vi "Agilent SNA Set Sweep Time.vi"(4 "Passthrough (T)":bool=TRUE, 6 "Channel":i8=1 min=1 max=99 step=1, 7 "Agilent SNA & SWP":T1, 8 "error in (no error)":errorcluster, 10 "Sweep Time, s (-1: Auto)":dbl=-1.0, 11 "VISA Resource Names":T2) -> (0 "error out":errorcluster, 3 "dup VISA Resource Names":T2)   [LabVIEW 2011]
doc: "This Vi for the HP8753B Network Analyzer is used to set averaging, smoothing, and the IF bandwidth."
uses:
  TypeDefs/Agilent SNA VISA.ctl
  TypeDefs/Agilent SNA Instrument Info.ctl
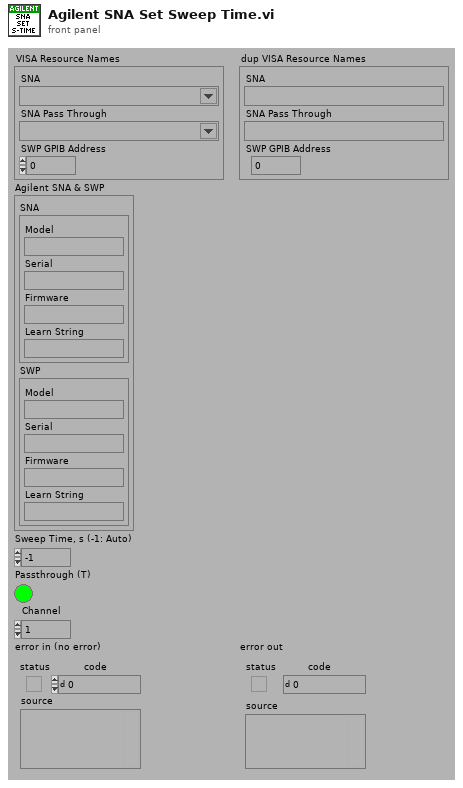
[diagram p1: front panel]
types:
  T1 = typedef "Agilent SNA Instrument Info.ctl" = cluster{"SNA":cluster{"Model":string, "Serial":string, "Firmware":string, "Learn String":string}, "SWP":cluster{"Model":string, "Serial":string, "Firmware":string, "Learn String":string}}
  T2 = typedef "Agilent SNA VISA.ctl" = cluster{"SNA":refnum<visa-resource-name>, "SNA Pass Through":refnum<visa-resource-name>, "SWP GPIB Address":i32}
  T3 = typedef "Agilent SNA Model.ctl" = enum16{"Not Supported", "8757X"}
  T4 = typedef "Agilent SNA SWP Model.ctl" = enum16{"Not Supported", "836XXX", "8375XX", "E82X7D"}
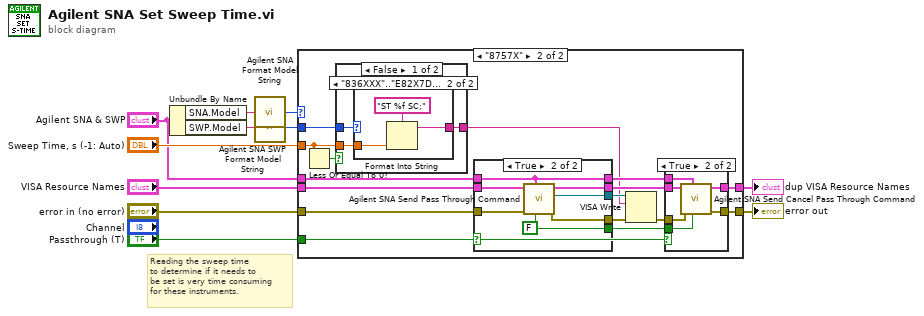
[diagram p0: block diagram]
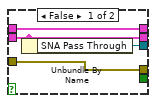
[diagram p4: hidden frame]
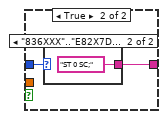
[diagram p6: hidden frame]
diagram:
  # "Reading the sweep time\nto determine if it needs to\nbe set is very time consuming\nfor these instruments."
  n1 = Unbundle By Name("Agilent SNA & SWP") -> ("SNA.Model"=w9:string, "SWP.Model"=w6:string)
  n2 = call "Agilent SNA Format Model String.vi"("Model String"=w9) -> ("Model"=w8:T3)
  n3 = call "Agilent SNA SWP Format Model String.vi"("Model String"=w6) -> ("Model"=w5:T4)
  n4 = case shown="\"8757X\"" w8 {
    tunnel: [w13 w17] -> w11
    tunnel: "error in (no error)" -> [w13 w20]
    tunnel: "Sweep Time, s (-1: Auto)" -> [_ w29]
    tunnel: "Agilent SNA & SWP" -> [_ w16]
    tunnel: w5 -> [_ w27]
    tunnel: [w12 w18] -> w3
    tunnel: "VISA Resource Names" -> [w12 w19]
    tunnel: "Passthrough (T)" -> [_ w14]
    frame "Not Supported" {
    }
    frame "8757X" {
      n5 = Less Or Equal To 0?(x=w29) -> (x <= 0?=w28:bool)
      n6 = case shown="False" w28 {
        tunnel: w29 -> [w51 _]
        tunnel: [w50 w56] -> w15
        tunnel: w27 -> [w49 w55]
        frame False {
          n7 = case shown="\"836XXX\"..\"E82X7D\"" w49 {
            tunnel: w51 -> [_ w53]
            tunnel: [_ w52] -> w50
            frame "Not Supported" {
            }
            frame "836XXX".."E82X7D" {
              n8 = Format Into String(format string="ST %f SC;", w53) -> (resulting string=w52:string)  [unwired: 2 in, 1 out]
            }
          }
        }
        frame True {
          n9 = case shown="\"836XXX\"..\"E82X7D\"" w55 {
            tunnel: [_ "ST 0 SC;"] -> w56
            frame "Not Supported" {
            }
            frame "836XXX".."E82X7D" {
            }
          }
        }
      }
      n10 = case shown="True" w14 {
        tunnel: [w39 w48] -> w25
        tunnel: w20 -> [w40 w47]
        tunnel: w19 -> [w38 w46]
        tunnel: [w40 w45] -> w23
        tunnel: w16 -> [w41 w42]
        tunnel: [w38 w44] -> w22
        tunnel: [_ w43] -> w26
        tunnel: [w41 w42] -> w21
        frame False {
          n11 = Unbundle By Name(w38) -> ("SNA Pass Through"=w39:refnum<visa-resource-name>)
        }
        frame True {
          w43 = FALSE ("SCPI? (F)")
          n12 = call "Agilent SNA Send Pass Through Command.vi"("SCPI? (F)"=w43, "Agilent SNA & SWP"=w42, "error in (no error)"=w47, "VISA Resource Names"=w46) -> ("error out"=w45:errorcluster, "SNA Pass Through"=w48:refnum<visa-resource-name>, "dup VISA Resource Names"=w44:T2)  [unwired: 5 out]
        }
      }
      n13 = VISA Write(VISA resource name=w25, write buffer=w15, error in (no error)=w23) -> (error out=w24:errorcluster)  [unwired: 2 out]
      n14 = case shown="True" w14 {
        tunnel: [w31 w37] -> w17
        tunnel: w22 -> [w30 w36]
        tunnel: w24 -> [w31 w35]
        tunnel: w26 -> [_ w34]
        tunnel: [w30 w33] -> w18
        tunnel: w21 -> [_ w32]
        frame False {
        }
        frame True {
          n15 = call "Agilent SNA Send Cancel Pass Through Command.vi"("SCPI? (F)"=w34, "Agilent SNA & SWP"=w32, "error in (no error)"=w35, "VISA Resource Names"=w36) -> ("error out"=w37:errorcluster, "dup VISA Resource Names"=w33:T2)  [unwired: 6 out]
        }
      }
    }
  }
  "error out" <- w11
  "dup VISA Resource Names" <- w3
